vi "Stop Video-reinitiate imaq.vi"(5 "Camera Fr":u16, 7 "Trigger Type":enum16{"Internal", "External"}(ring)=enum."External", 8 "error in":errorcluster, 9 "Frame Buffers In":T1[](array[typedef]), 11 "IMAQ Session In":refnum<k11>) -> (0 "error out":errorcluster)   [LabVIEW 2013]
uses:
  <vilib>/vision/Image Controls.llb/IMAQ Image.ctl
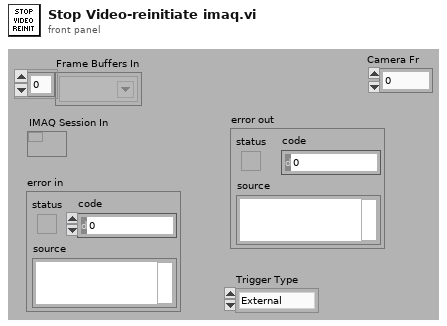
[diagram p1: front panel]
types:
  T1 = typedef "IMAQ Image.ctl" = refnum<image>
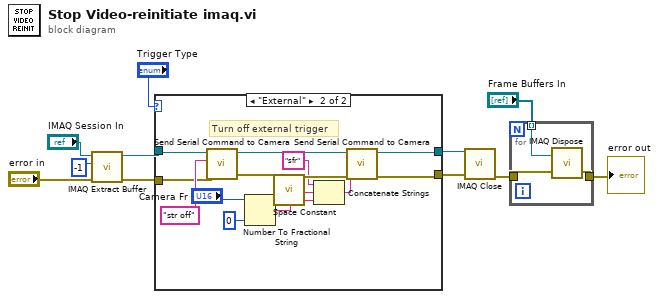
[diagram p0: block diagram]
diagram:
  n1 = call <vilib>:"IMAQ Extract Buffer.vi"("error in (no error)"="error in", "Buffer to extract"=-1, "IMAQ Session In"="IMAQ Session In") -> ("error out"=w5:errorcluster, "IMAQ Session Out"=w6:refnum<k11>)  [unwired: 3 in, 4 out]
  n2 = case shown="\"External\"" "Trigger Type" {
    tunnel: w6 -> [w13 w18]
    tunnel: w5 -> [w12 w17]
    tunnel: [w12 w15] -> w3
    tunnel: [w13 w16] -> w4
    frame "Internal", Default {
    }
    frame "External" {
      # "Turn off external trigger"
      n3 = call "Send Serial Command to Camera.vi"("error in (no error)"=w17, "String to write"="str off", "IMAQ Session In"=w18) -> ("error out"=w26:errorcluster, "IMAQ Session Out"=w25:refnum<k11>)  [unwired: 5 in, 2 out]
      n4 = Number To Fractional String(number="Camera Fr", precision (6)=i16 0) -> (F-format string=w22:string)  [unwired: 2 in]
      n5 = call <vilib>:"Space Constant.vi"() -> ("String"=w21:string)
      n6 = Concatenate Strings("sfr" ("string"), w21, w22) -> (w24:string)
      n7 = call "Send Serial Command to Camera.vi"("error in (no error)"=w26, "String to write"=w24, "IMAQ Session In"=w25) -> ("error out"=w15:errorcluster, "IMAQ Session Out"=w16:refnum<k11>)  [unwired: 5 in, 2 out]
    }
  }
  n8 = call <vilib>:"IMAQ Close.vi"("error in (no error)"=w3, "IMAQ Session In"=w4) -> ("error out"=w9:errorcluster)  [unwired: 9 in]
  n9 = for {
    tunnel: [w29] -> w7
    tunnel: w9 -> [w27]
    tunnel: "Frame Buffers In" -> [w28] mode=indexing
    n10 = call "IMAQ Dispose"("Image"=w28, "error in (no error)"=w27) -> ("error out"=w29:errorcluster)  [unwired: 4 in]
  }
  "error out" <- w7
